vi "Examen_U1_IVA.vi"() -> ()   [LabVIEW 2020]
uses:
  <vilib>/Instr/_visa.llb/VISA Configure Serial Port (Instr).vi
  <vilib>/express/express shared/transition.llb/Dynamic To Waveform Array.vi
  <vilib>/express/express signal manip/GetorSetDDTAttributes/Set DDT Attributes/SetT0.vi
  <vilib>/express/express shared/transition.llb/Waveform Array To Dynamic.vi
  <vilib>/express/express signal manip/GetorSetDDTAttributes/Set DDT Attributes/Set DDT Properties.xnode
panel:
  out "Graficando valores":bool
  out "Voltaje":i32
  out "Sensor":string
  out "Valor actual (Cm)":dbl
  out "Señal Original & Filtrada":dynamicdata(graph)
  out "Valor minimo (Cm)":i32
  out "Valor maximo (Cm)":i32
  in  "Selección Tarjeta":string(combo)="Arduino Mega"
  in  "?":bool
  out "Dato enviado":bool
  out "Tarjeta aceptada":bool
  out "Tarjeta a aceptar":string
  in  "Selección Puerto":refnum<visa-resource-name>
  # "Examen 01 - Instrumentación Virtual Aplicada\n\"Adquisición y análisis de señales analógicas y digitales con tarjeta de adquisición de datos\""
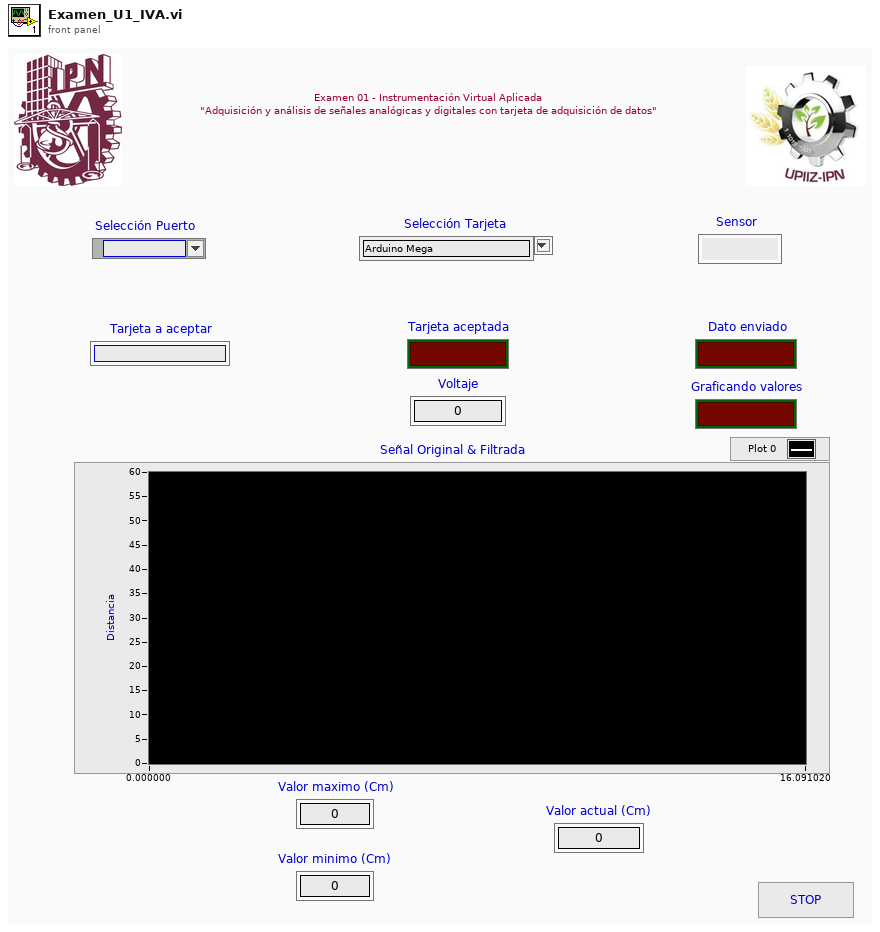
[diagram p1: front panel]
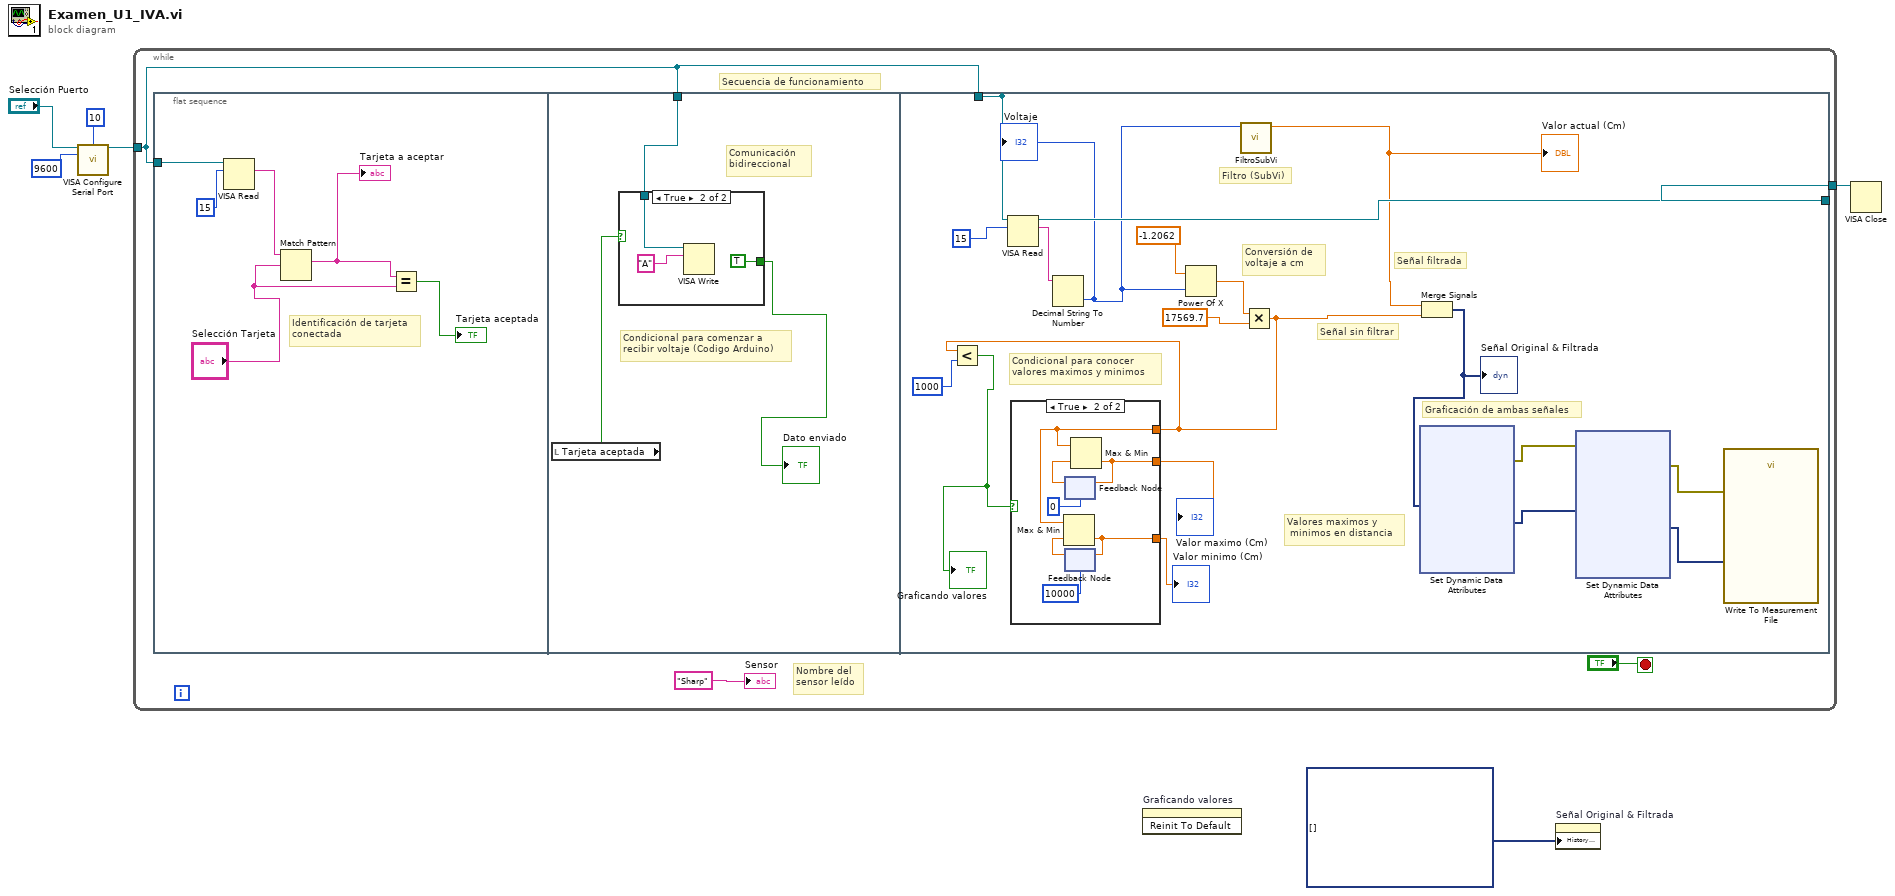
[diagram p0: block diagram]
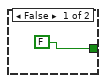
[diagram p2: hidden frame]
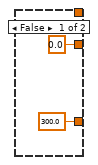
[diagram p3: hidden frame]
diagram:
  n1 = call-poly "VISA Configure Serial Port"("VISA resource name"="Selección Puerto", "termination char\n(0xA = '\\n' = LF)"=u8 10 ("termination char\n(0xA = '\\n' = LF)"), "baud rate (9600)"=u32 9600) -> ("VISA resource name out"=w3:refnum<visa-resource-name>)  [unwired: 11 in, 1 out]
  n2 = while {
    tunnel: w3 -> [w8]
    tunnel: [w9] -> w2
    stop <- "?" stop-if-true
    # "Secuencia de funcionamiento"
    # "Nombre del \nsensor leído"
    n3 = flat-sequence {
      tunnel: w8 -> [w15]
      tunnel: w8 -> [w17]
      tunnel: [w35] -> w9
      tunnel: [w33] -> _
      tunnel: w8 -> [w33]
      frame #0 {
        # "Identificación de tarjeta \nconectada"
        n4 = VISA Read(VISA resource name=w15, byte count=u32 15) -> (read buffer=w14:string)  [unwired: 1 in, 3 out]
        n5 = Match Pattern(string=w14, regular expression="Selección Tarjeta") -> (match substring=w13:string)  [unwired: 1 in, 3 out]
        "Tarjeta a aceptar" <- w13
        n6 = Equal?(x=w13, y="Selección Tarjeta") -> (x = y?=→"Tarjeta aceptada":bool)
      }
      frame #1 {
        # "Condicional para comenzar a \nrecibir voltaje (Codigo Arduino)"
        # "Comunicación \nbidireccional"
        n7 = local read "Tarjeta aceptada"() -> (w19:bool)
        n8 = case shown="True" w19 {
          tunnel: w17 -> [_ w22]
          tunnel: [FALSE TRUE] -> w18
          frame False {
          }
          frame True {
            n9 = VISA Write(VISA resource name=w22, write buffer="A") -> ()  [unwired: 1 in, 3 out]
          }
        }
        "Dato enviado" <- w18
      }
      frame #2 {
        # "Señal filtrada"
        # "Señal sin filtrar"
        # "Graficación de ambas señales"
        # "Conversión de \nvoltaje a cm"
        # "Filtro (SubVi)"
        # "Condicional para conocer \nvalores maximos y minimos"
        # "Valores maximos y\n minimos en distancia"
        n10 = VISA Read(VISA resource name=w33, byte count=u32 15) -> (VISA resource name out=w35:refnum<visa-resource-name>, read buffer=w41:string)  [unwired: 1 in, 2 out]
        n11 = Decimal String To Number(string=w41) -> (number=w30:i32)  [unwired: 2 in, 1 out]
        "Voltaje" <- w30
        n12 = Power Of X(1:w30, 2:-1.2062 ("x")) -> (0:w37:dbl)
        n13 = call "FiltroSubVi.vi"("Numeric in"=w30) -> ("Numeric"=w32:dbl)  [unwired: 10 in]
        "Valor actual (Cm)" <- w32
        n14 = Multiply(x=w37, y=17569.7) -> (x*y=w31:dbl)
        n15 = Less?(x=w31, y=1000) -> (x < y?=w29:bool)
        "Graficando valores" <- w29
        n16 = case shown="True" w29 {
          tunnel: [0.0 w75] -> w40
          tunnel: [300.0 w74] -> w39
          tunnel: w31 -> [_ w73]
          frame False {
          }
          frame True {
            n17 = feedback #1(0) -> (w79:dbl)
            n18 = feedback #2(10000) -> (w78:dbl)
            n19 = Max & Min(x=w73, y=w78) -> (min(x,y)=w74:dbl)  [unwired: 1 out]
            n20 = feedback-in #2(w74) -> ()
            n21 = Max & Min(x=w73, y=w79) -> (max(x,y)=w75:dbl)  [unwired: 1 out]
            n22 = feedback-in #1(w75) -> ()
          }
        }
        "Valor maximo (Cm)" <- w40
        "Valor minimo (Cm)" <- w39
        n23 = Merge Signals(w32, w31) -> (w24:dynamicdata)
        "Señal Original & Filtrada" <- w24
        n24 = xnode "Set Dynamic Data Attributes"("Signals In"=w24) -> ("Signals Out"=w28:dynamicdata, "error out"=w26:errorcluster)  [unwired: 3 in]
        n25 = xnode "Set Dynamic Data Attributes"("Signals In"=w28, "error in"=w26) -> ("Signals Out"=w27:dynamicdata, "error out"=w25:errorcluster)  [unwired: 2 in]
        n26 = call "Write To Measurement File"("Signals"=w27, "error in (no error)"=w25) -> ()  [unwired: 15 in, 3 out]
      }
    }
    "Sensor" <- "Sharp" ("read buffer 3")
  }
  n27 = invoke on="Graficando valores" class="Bool (strict)" method="Reinit To Default"() -> ()  [unwired: 3 in, 3 out]
  n28 = property on="Señal Original & Filtrada" class="WFChart (strict)"("History Data"=dynamicdata[] []) -> ()  [unwired: 2 in, 2 out]
  n29 = VISA Close(VISA resource name=w2) -> ()  [unwired: 1 in, 1 out]
